vi "Read Tree Items.vi"(11 "Test Tree In":refnum<class "Test Tree.lvclass">) -> (2 "Tree Items":T1(c390), 3 "Test Tree Out":refnum<class "Test Tree.lvclass">)   [LabVIEW 2020, in "Test Tree.lvclass"]
uses:
  Test Tree.lvclass
  Test Tree.lvclass/Test Tree.ctl
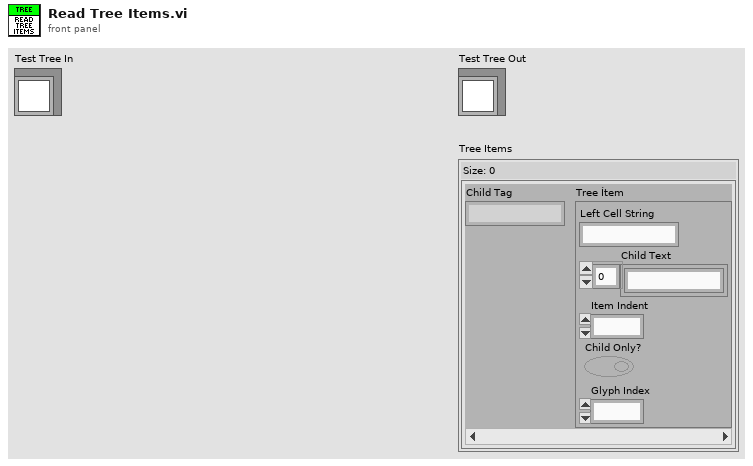
[diagram p1: front panel]
types:
  T1 = map{string, cluster{"Left Cell String":string, "Child Text":string[], "Item Indent":i32, "Child Only?":bool, "Glyph Index":i32}}
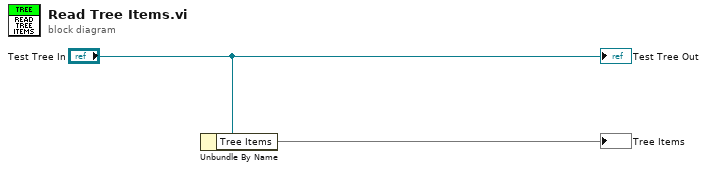
[diagram p0: block diagram]
diagram:
  n1 = Unbundle By Name("Test Tree In") -> ("Tree Items"=→"Tree Items":T1)
  "Test Tree Out" <- "Test Tree In"
